vi "Sample.vi"(8 "error in (no error)":errorcluster, 11 "Message Queues out":T1) -> (0 "error out":errorcluster, 3 "Message Queue":refnum<queue>)   [LabVIEW 2014]
uses:
  support/Message Queue/All Message Queues.ctl
  support/Message Queue/Message Cluster.ctl
  Sample data cluster.ctl
  Engine/Message.ctl
  Teszt/Teszt.ctl
  Teszt/Command.ctl
  support/Message Queue/Enqueue Message (Single).vi
  <vilib>/Utility/error.llb/Error Cluster From Error Code.vi
  support/Message Queue/Lossy Enqueue Message (Single).vi
  <vilib>/ErrorRing/Error Ring.xnode
  support/Message Queue/Message Queue.lvlib
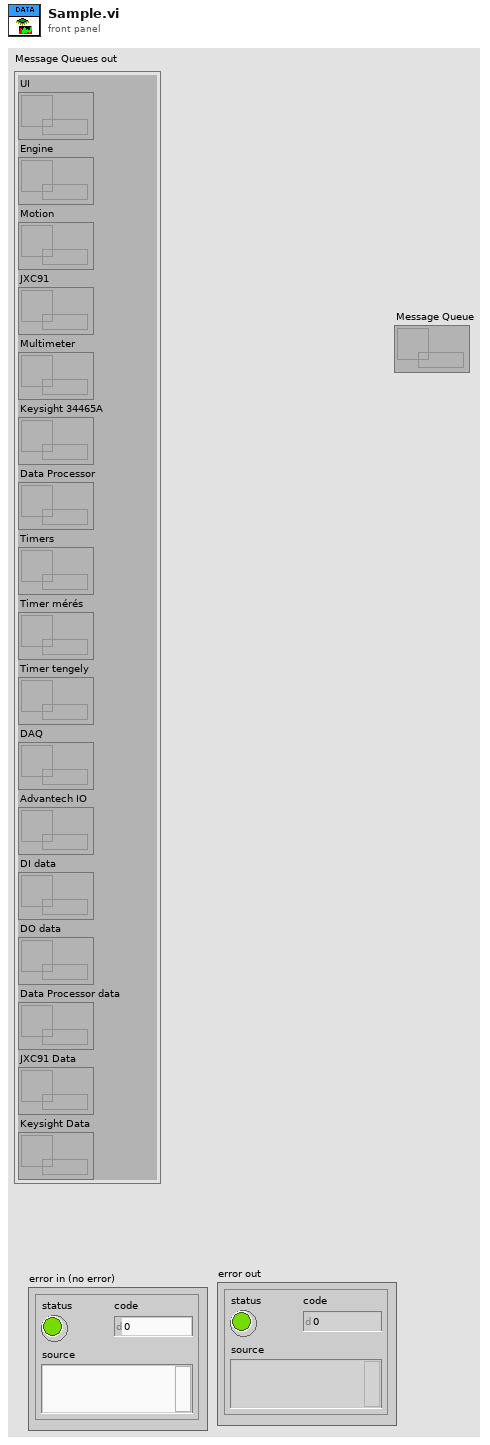
[diagram p1: front panel]
types:
  T1 = typedef "Message Queue.lvlib/All Message Queues.ctl" = cluster{"UI":refnum<queue>, "Engine":refnum<queue>, "Motion":refnum<queue>, "JXC91":refnum<queue>, "Multimeter":refnum<queue>, "Keysight 34465A":refnum<queue>, "Data Processor":refnum<queue>, "Timers":refnum<queue>, "Timer mérés":refnum<queue>, "Timer tengely":refnum<queue>, "DAQ":refnum<queue>, "Advantech IO":refnum<queue>, "DI data":refnum<queue>, "DO data":refnum<queue>, "Data Processor data":refnum<queue>, "JXC91 Data":refnum<queue>, "Keysight Data":refnum<queue>}
  T2 = typedef "Sample data cluster.ctl" = cluster{"Dummy":bool}
  T3 = typedef "Teszt.ctl" = cluster{"Thread ID":dbl, "Mérésszám":string, "Mérés/Utasítás":string, "Command":T4, "Min":string, "Max":string, "Aktív?":bool, "Log?":bool, "Kiértékelés":bool, "Etalon 1 exp":bool, "Etalon 2 exp":bool, "Etalon 3 exp":bool, "Etalon 4 exp":bool, "Etalon 5 exp":bool}
  T4 = typedef "Command.ctl" = cluster{"Parancs":string, "Paraméter 1":string, "Paraméter 2":string, "Paraméter 3":string, "Paraméter 4":string, "Paraméter 5":string, "Eredmény":string}
  T5 = typedef "Message.ctl" = cluster{"Thread ID":u16, "Callback":string, "Data":variant, "Error":errorcluster}
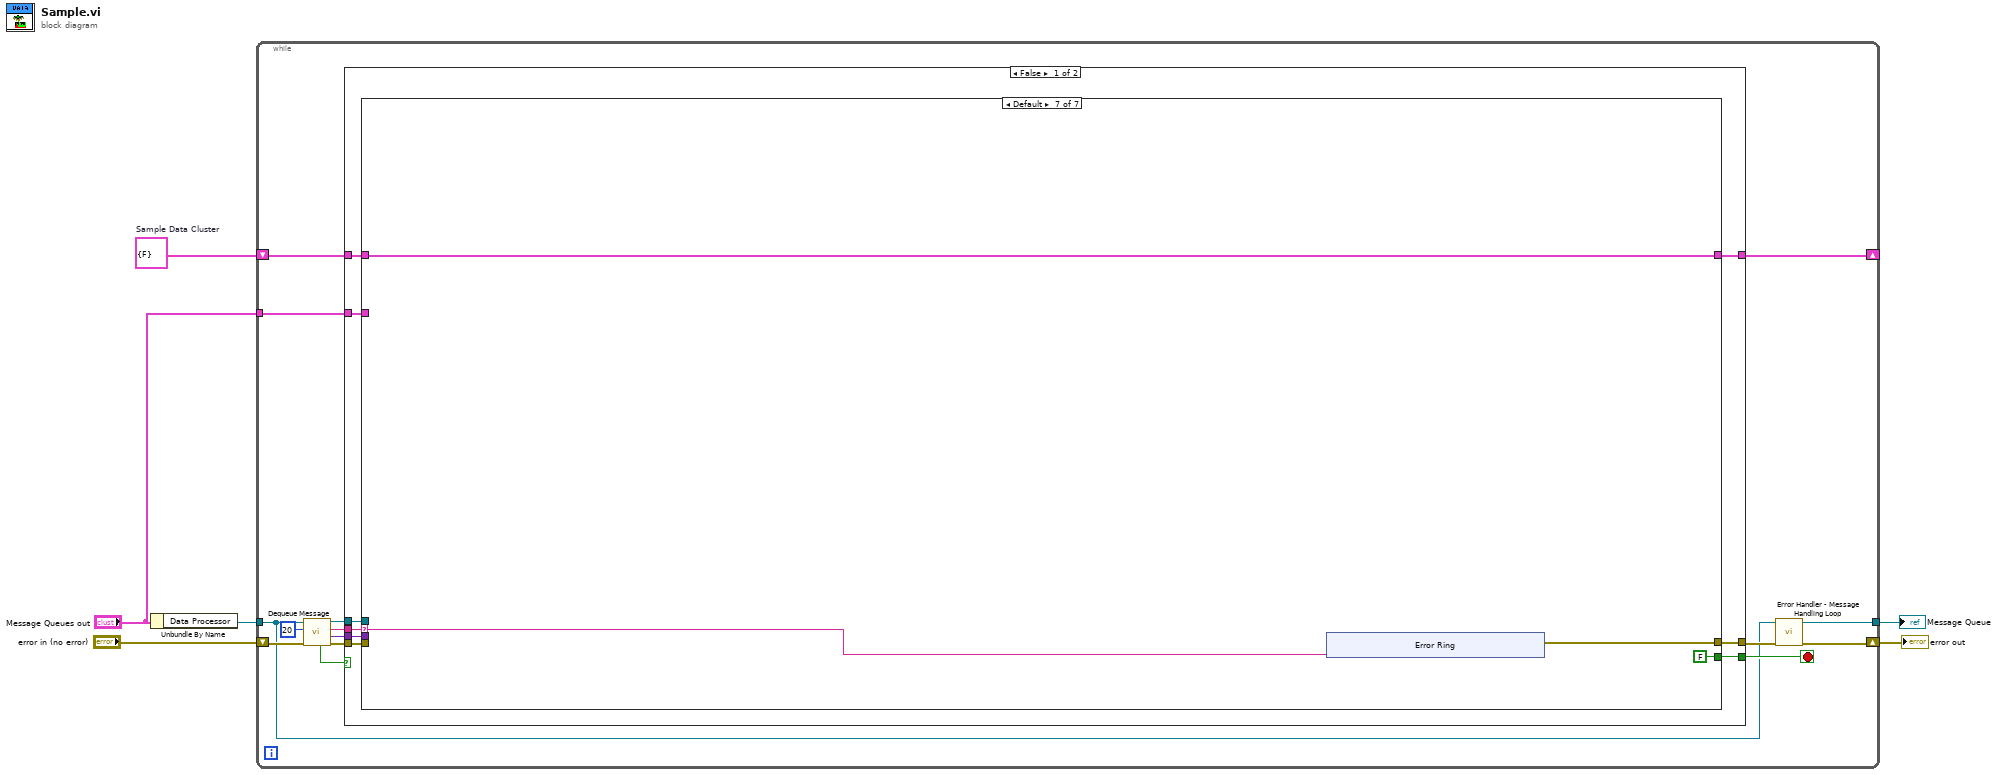
[diagram p0: block diagram]
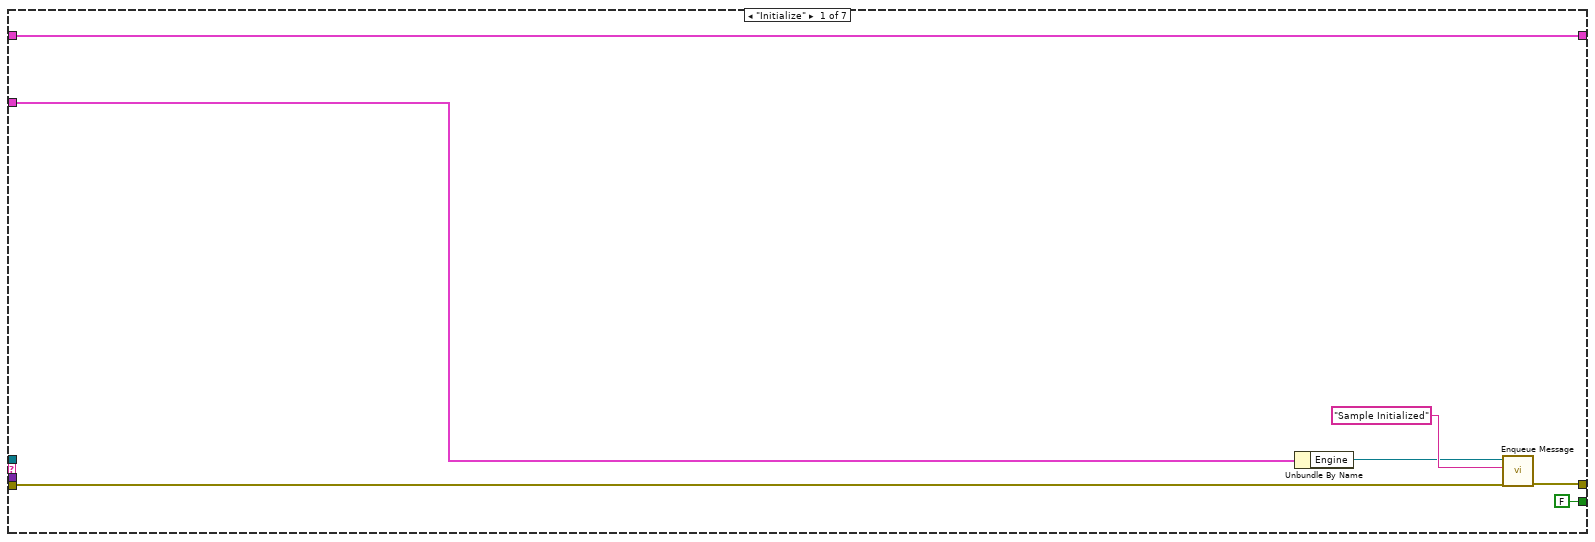
[diagram p2: hidden frame]
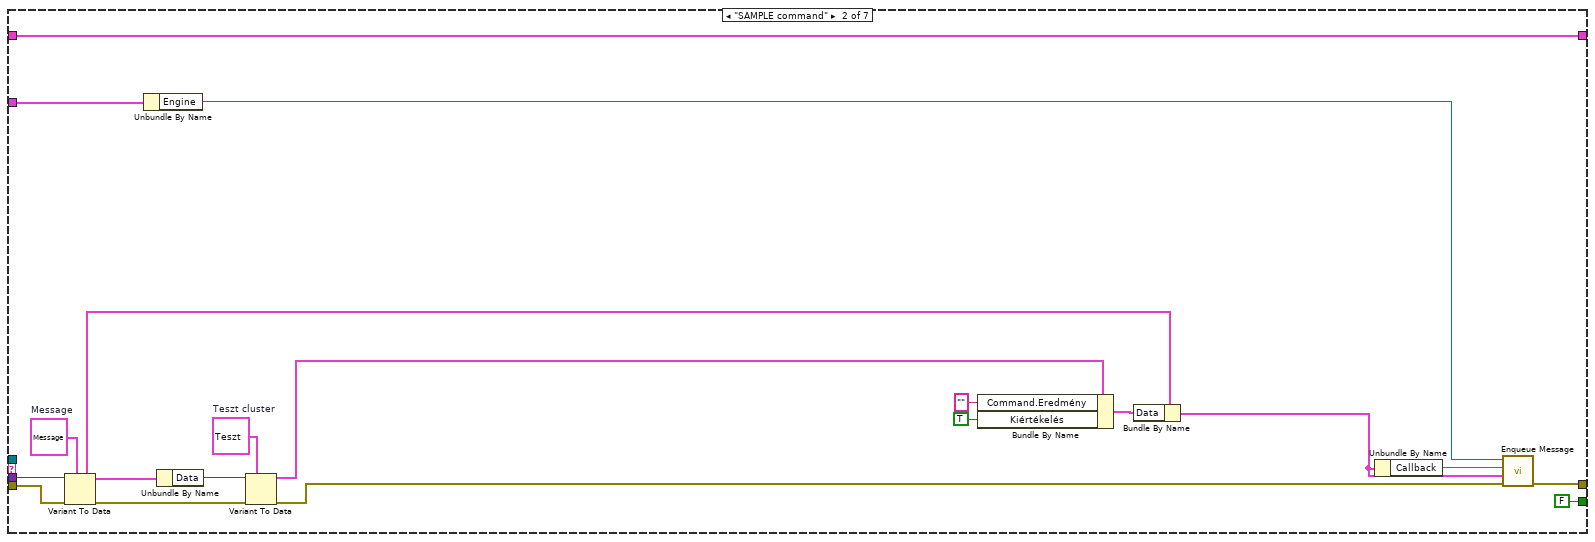
[diagram p3: hidden frame]
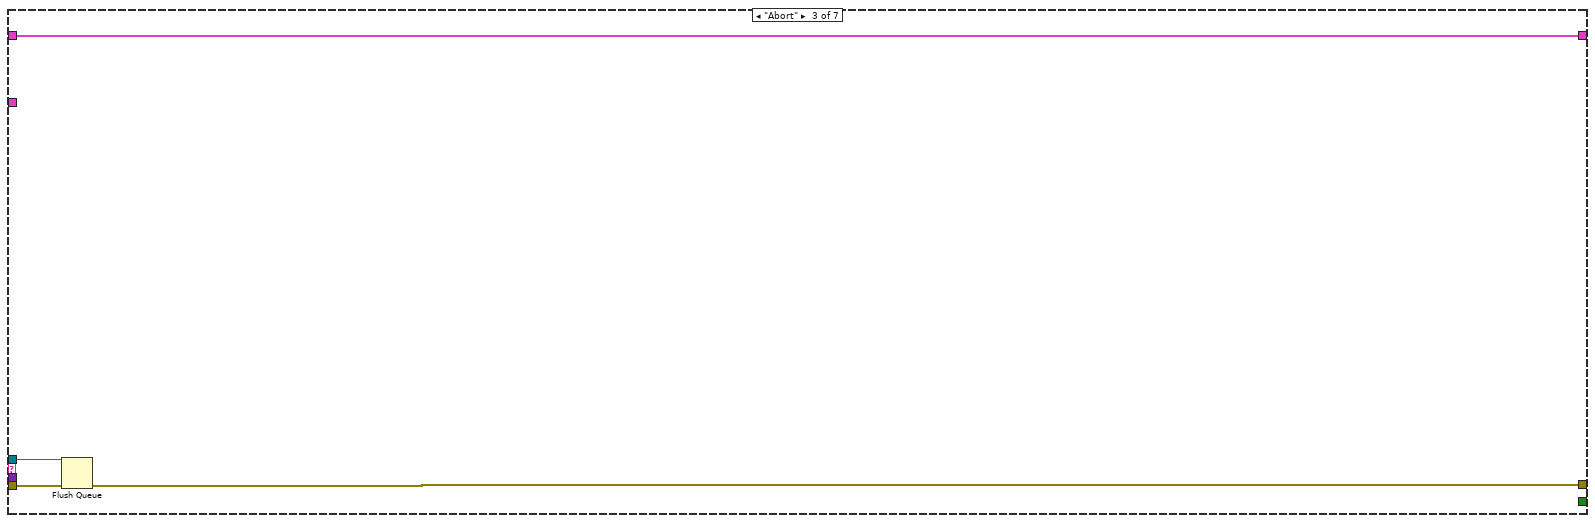
[diagram p4: hidden frame]
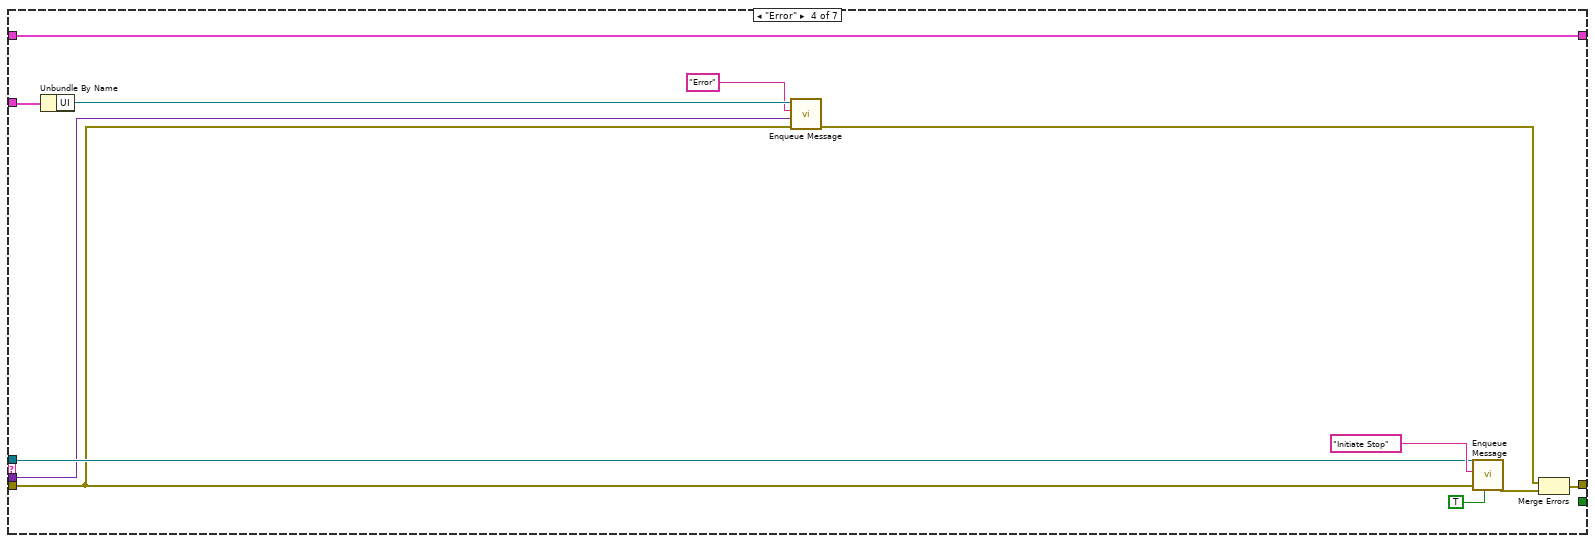
[diagram p5: hidden frame]
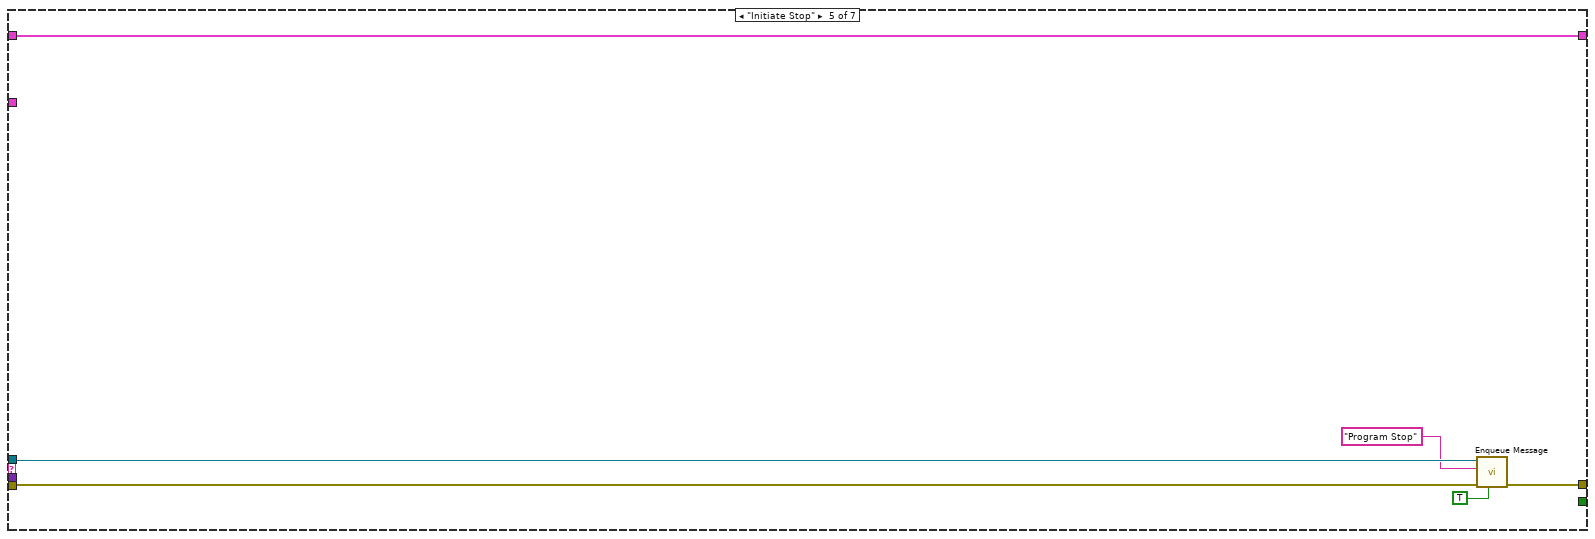
[diagram p6: hidden frame]
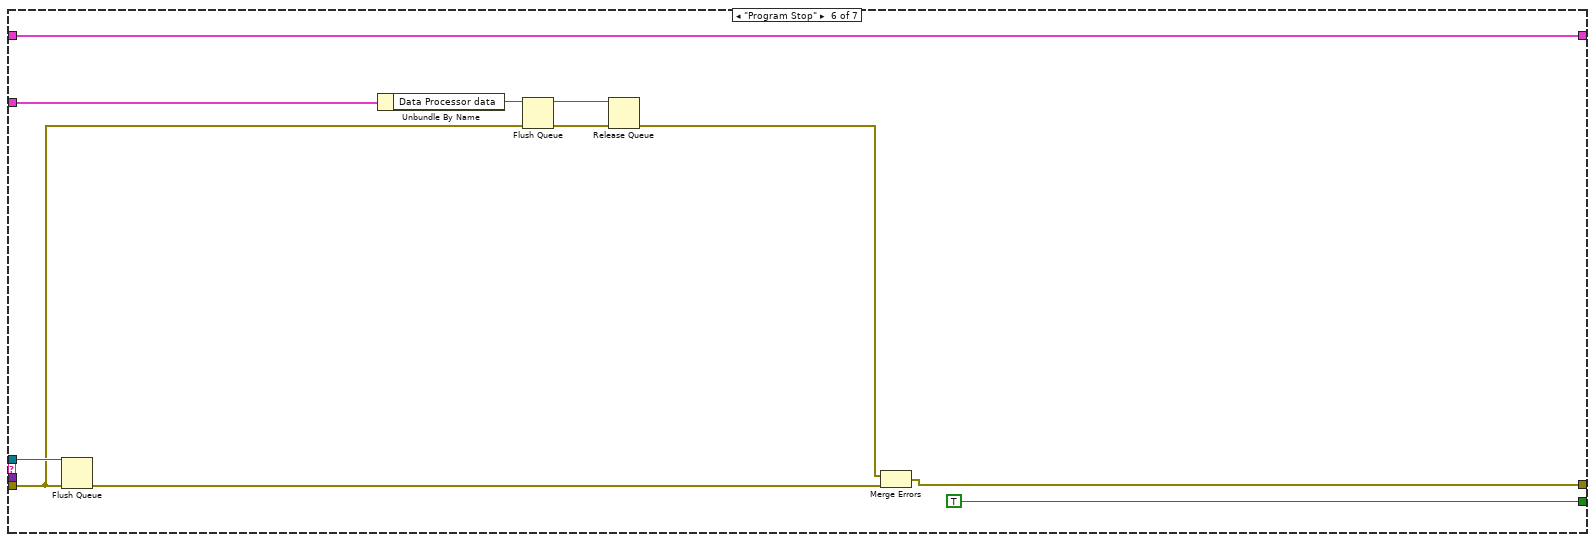
[diagram p7: hidden frame]
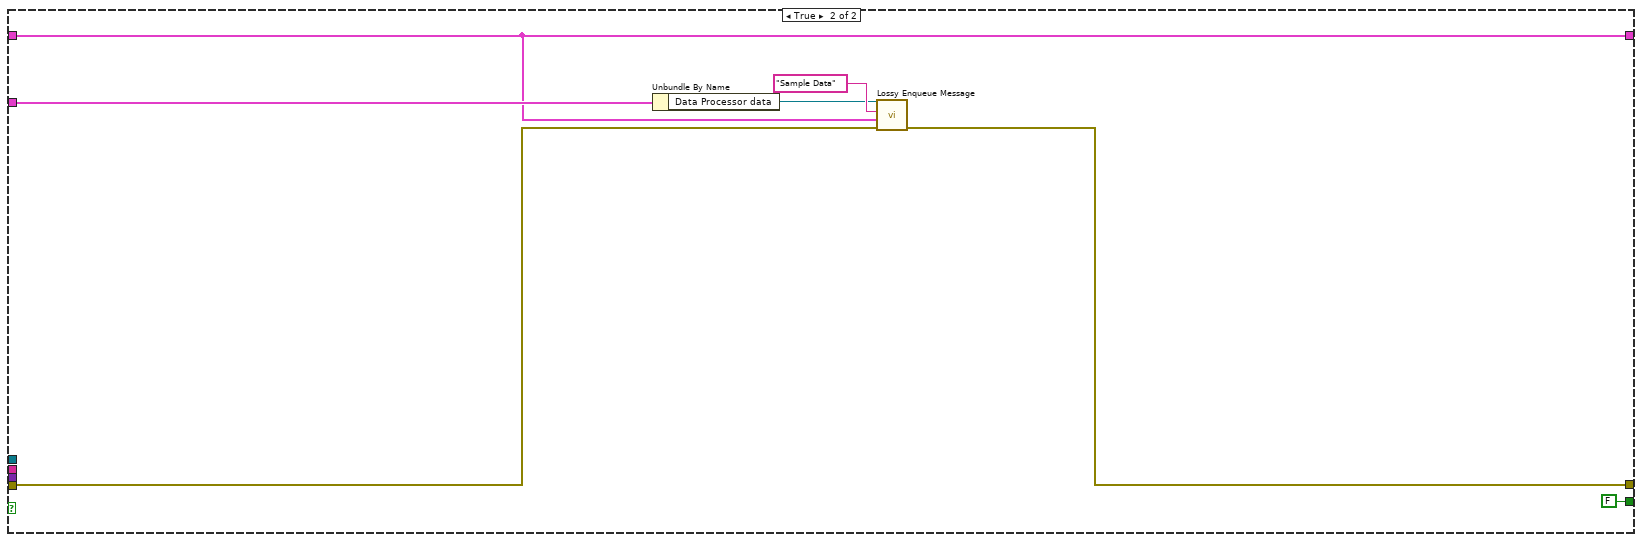
[diagram p8: hidden frame]
diagram:
  w1 = T2 {"Dummy"=FALSE}  # Sample Data Cluster
  n1 = Unbundle By Name("Message Queues out") -> ("Data Processor"=w3:refnum<queue>)
  n2 = while {
    tunnel: w3 -> [w7]
    shift-right: [w8] -> _
    shift-left: w1 -> [w14]
    shift-right: [w12] -> w6
    shift-left: "error in (no error)" -> [w21]
    tunnel: "Message Queues out" -> [w10]
    tunnel: [w9] -> w2
    stop <- w17 stop-if-true
    n3 = call "Dequeue Message.vi"("error in (no error)"=w21, "timeout in ms (-1)"=20, "Message Queue"=w7) -> ("error out"=w19:errorcluster, "Message Data"=w13:variant, "Message"=w20:string, "dup Message Queue"=w18:refnum<queue>, "timed out?"=w15:bool)  [unwired: 4 in]
    n4 = case shown="False" w15 {
      tunnel: w20 -> [w30 _]
      tunnel: w19 -> [w29 w102]
      tunnel: w18 -> [w28 _]
      tunnel: [w27 FALSE] -> w17
      tunnel: [w26 w101] -> w11
      tunnel: w14 -> [w24 w103]
      tunnel: [w25 w103] -> w8
      tunnel: w13 -> [w23 _]
      tunnel: w10 -> [w22 w104]
      frame False {
        n5 = case shown="Default" w30 {
          selector: w30 -> [_ _ _ _ _ _ w90]
          tunnel: w29 -> [w32 w48 w60 w62 w76 w79 _]
          tunnel: w28 -> [_ _ w59 w65 w75 w89 _]
          tunnel: [w36 w55 w57 w66 w77 w80 w91] -> w26
          tunnel: [FALSE FALSE _ _ _ TRUE FALSE] -> w27
          tunnel: [w31 w38 w58 w61 w78 w87 w93] -> w25
          tunnel: w24 -> [w31 w38 w58 w61 w78 w87 w93]
          tunnel: w23 -> [_ w47 _ w63 _ _ _]
          tunnel: w22 -> [w33 w53 _ w64 _ w82 _]
          frame "Initialize" {
            n6 = Unbundle By Name(w33) -> ("Engine"=w34:refnum<queue>)
            n7 = call-poly "Enqueue Message.vi"("error in (no error)"=w32, "Message"="Sample Initialized", "Message Queue"=w34) -> ("error out"=w36:errorcluster)  [unwired: 7 in, 1 out]
          }
          frame "SAMPLE command" {
            w49 = T3 {"Thread ID"=0.0, "Mérésszám"="", "Mérés/Utasítás"="", "Command"={"Parancs"="", "Paraméter 1"="", "Paraméter 2"="", "Paraméter 3"="", "Paraméter 4"="", "Paraméter 5"="", "Eredmény"=""}, "Min"="", "Max"="", "Aktív?"=FALSE, "Log?"=FALSE, "Kiértékelés"=FALSE, "Etalon 1 exp"=FALSE, "Etalon 2 exp"=FALSE, "Etalon 3 exp"=FALSE, "Etalon 4 exp"=FALSE, "Etalon 5 exp"=FALSE}  # Teszt cluster
            w52 = T5 {"Thread ID"=0, "Callback"="", "Data"=variant, "Error"={"status"=FALSE, "code"=0, "source"=""}}  # Message
            n8 = Variant To Data(error in=w48, type=w52, Variant=w47) -> (data=w43:T5, error out=w51:errorcluster)
            n9 = Unbundle By Name(w53) -> ("Engine"=w54:refnum<queue>)
            n10 = Unbundle By Name(w43) -> ("Data"=w50:variant)
            n11 = Variant To Data(error in=w51, type=w49, Variant=w50) -> (data=w39:T3, error out=w42:errorcluster)
            n12 = Bundle By Name(cluster=w39, "Command.Eredmény"="", "Kiértékelés"=TRUE) -> (w46:T3)
            n13 = Bundle By Name(cluster=w43, "Data"=w46) -> (w44:T5)
            n14 = Unbundle By Name(w44) -> ("Callback"=w45:string)
            n15 = call-poly "Enqueue Message.vi"("error in (no error)"=w42, "Message Data"=w44, "Message"=w45, "Message Queue"=w54) -> ("error out"=w55:errorcluster)  [unwired: 6 in, 1 out]
          }
          frame "Abort" {
            n16 = Flush Queue(queue=w59, error in (no error)=w60) -> (error out=w57:errorcluster)  [unwired: 2 out]
          }
          frame "Error" {
            n17 = Unbundle By Name(w64) -> ("UI"=w69:refnum<queue>)
            n18 = call-poly "Enqueue Message.vi"("error in (no error)"=w62, "Message Data"=w63, "Message"="Error", "Message Queue"=w69) -> ("error out"=w71:errorcluster)  [unwired: 6 in, 1 out]
            n19 = call-poly "Enqueue Message.vi"("Priority Message? (F)"=TRUE, "error in (no error)"=w62, "Message"="Initiate Stop", "Message Queue"=w65) -> ("error out"=w70:errorcluster)  [unwired: 6 in, 1 out]
            n20 = Merge Errors(w71, w70) -> (w66:errorcluster)
          }
          frame "Initiate Stop" {
            n21 = call-poly "Enqueue Message.vi"("Priority Message? (F)"=TRUE, "error in (no error)"=w76, "Message"="Program Stop", "Message Queue"=w75) -> ("error out"=w77:errorcluster)  [unwired: 6 in, 1 out]
          }
          frame "Program Stop" {
            n22 = Flush Queue(queue=w89, error in (no error)=w79) -> (error out=w81:errorcluster)  [unwired: 2 out]
            n23 = Unbundle By Name(w82) -> ("Data Processor data"=w83:refnum<queue>)
            n24 = Flush Queue(queue=w83, error in (no error)=w79) -> (queue out=w84:refnum<queue>, error out=w85:errorcluster)  [unwired: 1 out]
            n25 = Release Queue(queue=w84, error in (no error)=w85) -> (error out=w86:errorcluster)  [unwired: 1 in, 2 out]
            n26 = Merge Errors(w86, w81) -> (w80:errorcluster)
          }
          frame Default {
            n27 = xnode "Error Ring"("parameter 0"=w90) -> ("error out"=w91:errorcluster)
          }
        }
      }
      frame True {
        n28 = Unbundle By Name(w104) -> ("Data Processor data"=w105:refnum<queue>)
        n29 = call-poly "Lossy Enqueue Message.vi"("error in (no error)"=w102, "Message Data"=w103, "Message"="Sample Data", "Message Queue"=w105) -> ("error out"=w101:errorcluster)  [unwired: 6 in, 1 out]
      }
    }
    n30 = call "Error Handler - Message Handling Loop.vi"("error in (no error)"=w11, "Message Queue"=w7) -> ("dup error in"=w12:errorcluster, "dup Message Queue"=w9:refnum<queue>)  [unwired: 8 in]
  }
  "error out" <- w6
  "Message Queue" <- w2
